vi "Display3DTest.vi"(8 "error in":errorcluster, 11 "Local":T7={"Parameter"={"3D Plot"=[], "3D Scatter"=refnum, "Data"={"Split"={"X Train"=[], "X Test"=[], "Y Train"=[], "Y Test"=[]}, "Predict"=[]}, "Display"={"Choice"=enum."All", "Indexe"={"X"=0, "Y"=1, "Z"=2}}, "Point Property"={"Train Style"=enum."Full circle", "Test OK Style"=enum."Full square", "Label Color"=[8978528, 4367871, 1985280], "Test NO OK"={"Style"=enum."Cross", "Color"=16716800}}, "3D Plot Datatype.lvclass"=refnum}, "3DArray"=[], "Rating 3D Array"=[], "GoodPredict"=0, "Point ID"=[]}) -> (0 "error out":errorcluster, 3 "Local Out":T5={"Parameter"={"3D Plot"=[], "3D Scatter"=refnum, "Data"={"Split"={"X Train"=[], "X Test"=[], "Y Train"=[], "Y Test"=[]}, "Predict"=[]}, "Display"={"Choice"=enum."All", "Indexe"={"X"=0, "Y"=1, "Z"=2}}, "Point Property"={"Train Style"=enum."Full circle", "Test OK Style"=enum."Full square", "Label Color"=[8978528, 4367871, 1985280], "Test NO OK"={"Style"=enum."Cross", "Color"=16716800}}, "3D Plot Datatype.lvclass"=refnum}, "3DArray"=[], "Rating 3D Array"=[], "GoodPredict"=0, "Point ID"=[]})   [LabVIEW 2020]
doc: "Display the 3D predicted data"
uses:
  _Controls/3DParameters.ctl
  <vilib>/Math Plots/3D Math Plots/3D Plot/3D Plot Datatype/3D Plot Datatype.lvclass
  <vilib>/Math Plots/3D Math Plots/3D Scatter/3D Scatter XCtrl/3D Scatter.xctl
  _Controls/Datas.ctl
  _Controls/PointPropertyMultipleLabel.ctl
  _Controls/Style.ctl
  _Controls/3DData.ctl
  <vilib>/Math Plots/3D Math Plots/3D Plot/3D Plot/Typedef/Color Ramp Cluster.ctl
  <vilib>/Math Plots/3D Math Plots/3D Plot/3D Plot/3D Plot.lvclass
types:
  T1 = typedef "Datas.ctl" = cluster{"Split":cluster{"X Train":dbl[][], "X Test":dbl[][], "Y Train":dbl[][], "Y Test":dbl[][]}, "Predict":dbl[][]}
  T2 = typedef "PointPropertyMultipleLabel.ctl" = cluster{"Train Style":T3, "Test OK Style":T3, "Label Color":u32[], "Test NO OK":cluster{"Style":T3, "Color":u32}}
  T3 = typedef "Style.ctl" = enum16{"Empty circle", "Full circle", "Empty square", "Full square", "Cross"}
  T4 = typedef "3DData.ctl" = cluster{"Tag":i32, "X":dbl[], "Y":dbl[], "Z":dbl[]}
  T5 = cluster{"Parameter":cluster{"3D Plot":refnum<class "3D Plot Datatype.lvclass">[], "3D Scatter":refnum<vi>, "Data":T1, "Display":cluster{"Choice":enum16{"All", "Train", "Test"}, "Indexe":cluster{"X":i32, "Y":i32, "Z":i32}}, "Point Property":T2, "3D Plot Datatype.lvclass":refnum<class "3D Plot Datatype.lvclass">}, "3DArray":cluster{"X":dbl[], "Y":dbl[], "Z":dbl[]}[], "Rating 3D Array":T4[], "GoodPredict":i32, "Point ID":cluster{"DataUse":enum16{"Dataset", "Train", "Test"}, "Color":u32}[]}
  T6 = typedef "3DParameters.ctl" = cluster{"3D Plot":refnum<class "3D Plot Datatype.lvclass">[], "3D Scatter":refnum<vi>, "Data":T1, "Display":cluster{"Choice":enum16{"All", "Train", "Test"}, "Indexe":cluster{"X":i32, "Y":i32, "Z":i32}}, "Point Property":T2, "3D Plot Datatype.lvclass":refnum<class "3D Plot Datatype.lvclass">}
  T7 = cluster{"Parameter":T6, "3DArray":cluster{"X":dbl[], "Y":dbl[], "Z":dbl[]}[], "Rating 3D Array":T4[], "GoodPredict":i32, "Point ID":cluster{"DataUse":enum16{"Dataset", "Train", "Test"}, "Color":u32}[]}
  T8 = typedef "3D Plot.lvclass/Color Ramp Cluster.ctl" = cluster{"Color Ramp Style":enum16{"None", "Shaded", "Color spectrum", "Grey scale", "Custom"}, "Color Ramp Array":u32[], "Color Ramp Index":i32[], "Interpolate?":bool, "Logarithm?":bool}
  T9 = typedef "3D Plot.lvclass/Sprite Type.ctl" = enum16{"None", "Empty Square", "Solid Square", "Empty Diamond", "Solid Diamond", "Empty Circle", "Solid Circle", "Asterisk", "Bold X", "Wireframe Sphere", "Solid Sphere", "Wireframe Cube", "Solid Cube"}
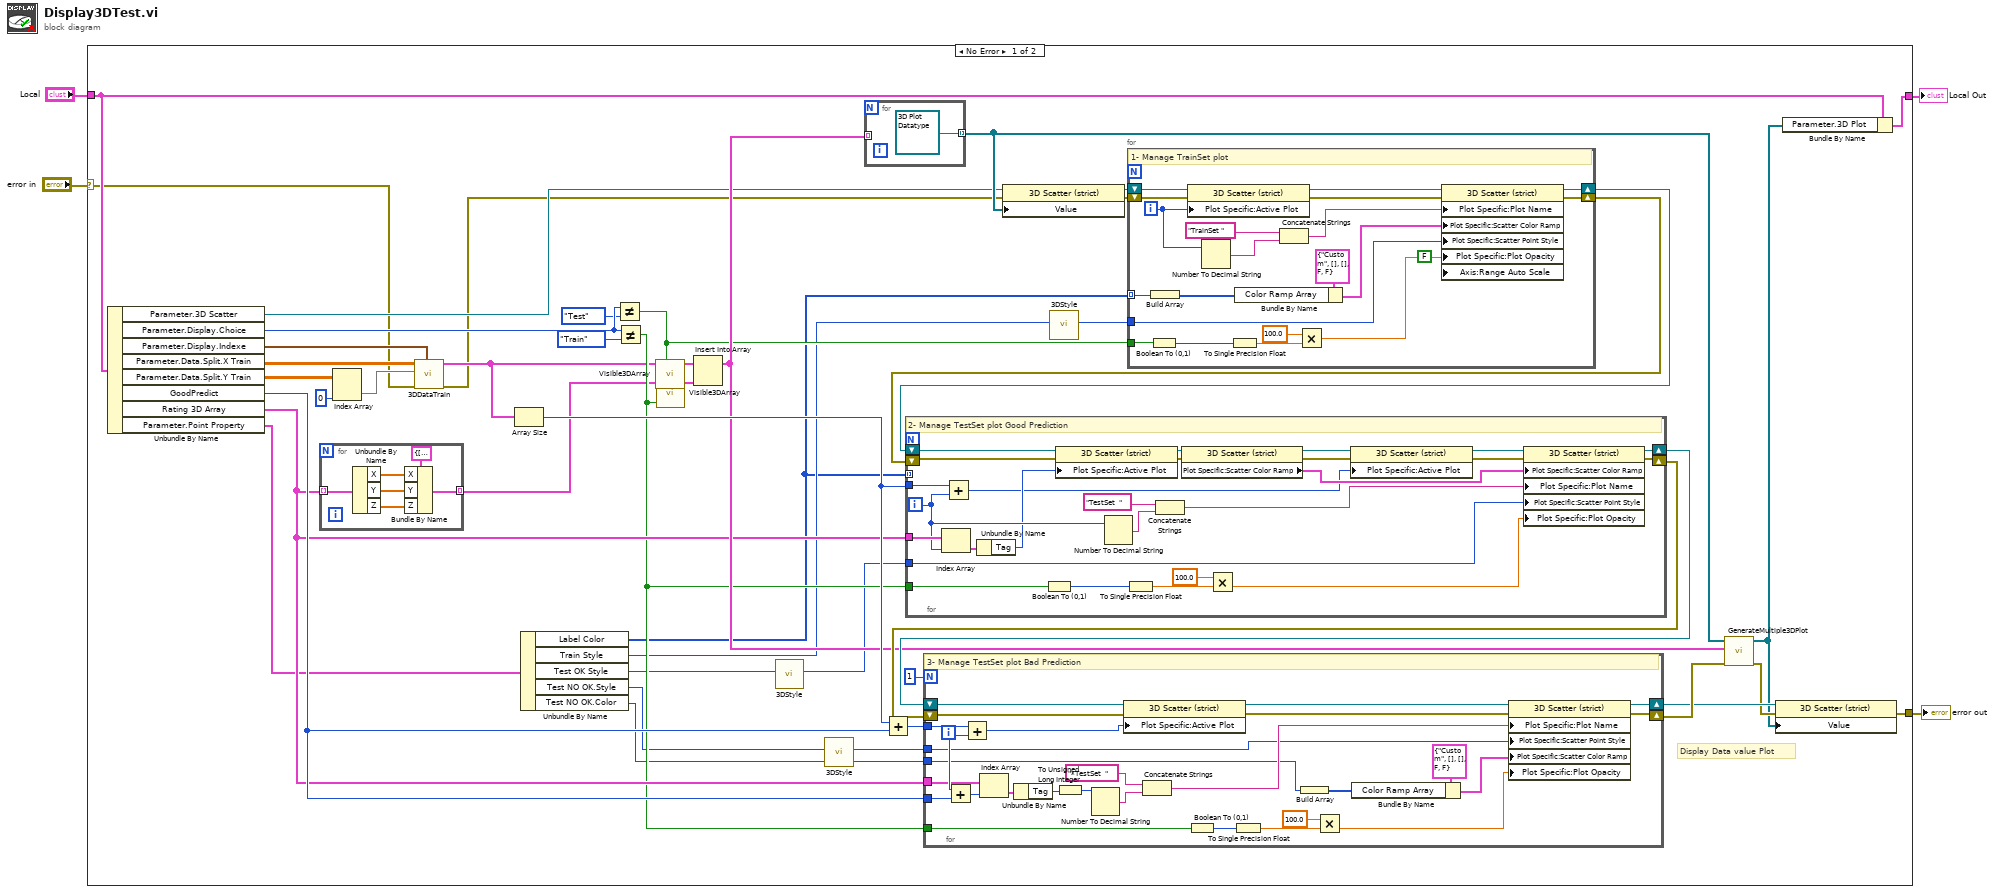
[diagram p0: block diagram]
diagram:
  n1 = case shown="No Error" "error in" {
    selector: "error in" -> [w15 w134]
    tunnel: [w28 w134] -> w3
    tunnel: "Local" -> [w39 w133]
    tunnel: [w38 w133] -> w1
    frame No Error {
      # "Display Data value Plot"
      n2 = Unbundle By Name(w39) -> ("Parameter.3D Scatter"=w32:refnum<vi>, "Parameter.Display.Choice"=w36:enum16{"All", "Train", "Test"}, "Parameter.Display.Indexe"=w16:cluster{"X":i32, "Y":i32, "Z":i32}, "Parameter.Data.Split.X Train"=w20:dbl[][], "Parameter.Data.Split.Y Train"=w35:dbl[][], "GoodPredict"=w34:i32, "Rating 3D Array"=w33:T4[], "Parameter.Point Property"=w14:T2)
      n3 = for {
        tunnel: w33 -> [w56] mode=indexing
        tunnel: [w54] -> w24 mode=indexing
        n4 = Unbundle By Name(w56) -> ("X"=w53:dbl[], "Y"=w52:dbl[], "Z"=w51:dbl[])
        n5 = Bundle By Name(cluster=cluster{"X":dbl[], "Y":dbl[], "Z":dbl[]} {"X"=[], "Y"=[], "Z"=[]} ("new element/subarray"), "X"=w53, "Y"=w52, "Z"=w51) -> (w54:cluster{"X":dbl[], "Y":dbl[], "Z":dbl[]})
      }
      n6 = Index Array(array=w35, index (col)=0 ("disabled index (col)")) -> (element=w19:dbl[])  [unwired: 1 in]
      n7 = call "3DDataTrain.vi"("Index"=w16, "error in"=w15, "Y"=w19, "X"=w20) -> ("error out"=w21:errorcluster, "3DArray"=w22:cluster{"X":dbl[], "Y":dbl[], "Z":dbl[]}[])  [unwired: 6 in]
      n8 = Array Size(array=w22) -> (size(s)=w42:i32)
      n9 = Unbundle By Name(w14) -> ("Label Color"=w8:u32[], "Train Style"=w10:T3, "Test OK Style"=w7:T3, "Test NO OK.Style"=w12:T3, "Test NO OK.Color"=w13:u32)
      n10 = Not Equal?(x=w36, y=enum16{"All", "Train", "Test"}."Test") -> (x != y?=w27:bool)
      n11 = Not Equal?(x=w36, y=enum16{"All", "Train", "Test"}."Train") -> (x != y?=w25:bool)
      n12 = call "Visible3DArray.vi"("Visible"=w27, "Array In"=w22) -> ("Array Out"=w26:cluster{"X":dbl[], "Y":dbl[], "Z":dbl[]}[])  [unwired: 9 in]
      n13 = call "Visible3DArray.vi"("Visible"=w25, "Array In"=w24) -> ("Array Out"=w23:cluster{"X":dbl[], "Y":dbl[], "Z":dbl[]}[])  [unwired: 9 in]
      n14 = Insert Into Array(array=w26, new element=w23) -> (w41:cluster{"X":dbl[], "Y":dbl[], "Z":dbl[]}[])  [unwired: 1 in]
      n15 = call "3DStyle.vi"("Style"=w7) -> ("Scatter Point Style"=w6:T9)  [unwired: 10 in]
      n16 = call "3DStyle.vi"("Style"=w12) -> ("Scatter Point Style"=w11:T9)  [unwired: 10 in]
      n17 = for {
        tunnel: w41 -> [_] mode=indexing
        tunnel: [refnum<class "3D Plot Datatype.lvclass"> refnum ("3D Plot Datatype.lvclass")] -> w37 mode=indexing
      }
      n18 = Add(x=w42, y=w34) -> (x+y=w46:i32)
      n19 = property class="3D Scatter (strict)"(reference=w32, error in=w21, "Value"=w37) -> (reference out=w44:refnum<vi>, error out=w43:errorcluster)
      n20 = call "3DStyle.vi"("Style"=w10) -> ("Scatter Point Style"=w9:T9)  [unwired: 10 in]
      n21 = for {
        shift-right: [w126] -> w50
        shift-left: w43 -> [w131]
        shift-right: [w125] -> w49
        shift-left: w44 -> [w132]
        tunnel: w27 -> [w123]
        tunnel: w8 -> [w115] mode=indexing
        tunnel: w9 -> [w112]
        i -> [w124]
        # "1- Manage TrainSet plot"
        n22 = Boolean To (0,1)(Boolean=w123) -> (0, 1=w122:i16)
        n23 = Build Array(w115) -> (w114:u32[])
        n24 = property class="3D Scatter (strict)"(reference=w132, error in=w131, "Plot Specific:Active Plot"=w124) -> (reference out=w130:refnum<vi>, error out=w129:errorcluster)
        n25 = Number To Decimal String(number=w124) -> (decimal integer string=w127:string)  [unwired: 1 in]
        n26 = To Single Precision Float(number=w122) -> (single precision float=w121:sgl)
        n27 = Bundle By Name(cluster=T8 {"Color Ramp Style"=enum."Custom", "Color Ramp Array"=[], "Color Ramp Index"=[], "Interpolate?"=FALSE, "Logarithm?"=FALSE} ("Spécifique à un tracé:Nuage:Rampe de couleur du nuage"), "Color Ramp Array"=w114) -> (w113:T8)
        n28 = Concatenate Strings("TrainSet " ("Plot.Plot Name"), w127) -> (w116:string)
        n29 = Multiply(x=sgl 100.0, y=w121) -> (x*y=w120:sgl)
        n30 = property class="3D Scatter (strict)"(reference=w130, error in=w129, "Plot Specific:Plot Name"=w116, "Plot Specific:Scatter Color Ramp"=w113, "Plot Specific:Scatter Point Style"=w112, "Plot Specific:Plot Opacity"=w120, "Axis:Range Auto Scale"=FALSE ("Axis:Range:Range Auto Scale")) -> (reference out=w125:refnum<vi>, error out=w126:errorcluster)
      }
      n31 = for {
        shift-right: [w68] -> w47
        shift-left: w50 -> [w73]
        shift-right: [w78] -> w48
        shift-left: w49 -> [w74]
        tunnel: w42 -> [w76]
        tunnel: w33 -> [w77]
        tunnel: w25 -> [w61]
        tunnel: w8 -> [_] mode=indexing
        tunnel: w6 -> [w57]
        i -> [w67]
        # "2- Manage TestSet plot Good Prediction"
        n32 = Index Array(array=w77, index=w67) -> (element=w75:T4)
        n33 = Add(x=w76, y=w67) -> (x+y=w63:i32)
        n34 = Unbundle By Name(w75) -> ("Tag"=w64:i32)
        n35 = Boolean To (0,1)(Boolean=w61) -> (0, 1=w62:i16)
        n36 = property class="3D Scatter (strict)"(reference=w74, error in=w73, "Plot Specific:Active Plot"=w64) -> (reference out=w72:refnum<vi>, error out=w71:errorcluster)
        n37 = Number To Decimal String(number=w67) -> (decimal integer string=w79:string)  [unwired: 1 in]
        n38 = To Single Precision Float(number=w62) -> (single precision float=w60:sgl)
        n39 = Concatenate Strings("TestSet  " ("Plot.Plot Name"), w79) -> (w66:string)
        n40 = property class="3D Scatter (strict)"(reference=w72, error in=w71) -> (reference out=w70:refnum<vi>, error out=w69:errorcluster, "Plot Specific:Scatter Color Ramp"=w65:T8)
        n41 = Multiply(x=sgl 100.0, y=w60) -> (x*y=w59:sgl)
        n42 = property class="3D Scatter (strict)"(reference=w70, error in=w69, "Plot Specific:Active Plot"=w63) -> (reference out=w82:refnum<vi>, error out=w81:errorcluster)
        n43 = property class="3D Scatter (strict)"(reference=w82, error in=w81, "Plot Specific:Scatter Color Ramp"=w65, "Plot Specific:Plot Name"=w66, "Plot Specific:Scatter Point Style"=w57, "Plot Specific:Plot Opacity"=w59) -> (reference out=w78:refnum<vi>, error out=w68:errorcluster)
      }
      n44 = for {
        N: 1 -> [_]
        shift-right: [w102] -> w40
        shift-left: w47 -> [w96]
        shift-right: [w106] -> w31
        shift-left: w48 -> [w95]
        tunnel: w46 -> [w105]
        tunnel: w33 -> [w99]
        tunnel: w34 -> [w100]
        tunnel: w25 -> [w90]
        tunnel: w13 -> [w84]
        tunnel: w11 -> [w83]
        i -> [w101]
        # "3- Manage TestSet plot Bad Prediction"
        n45 = Add(x=w101, y=w100) -> (x+y=w98:i32)
        n46 = Add(x=w105, y=w101) -> (x+y=w94:i32)
        n47 = Index Array(array=w99, index=w98) -> (element=w104:T4)
        n48 = Unbundle By Name(w104) -> ("Tag"=w103:i32)
        n49 = To Unsigned Long Integer(number=w103) -> (unsigned 32bit integer=w97:u32)
        n50 = Number To Decimal String(number=w97) -> (decimal integer string=w107:string)  [unwired: 1 in]
        n51 = property class="3D Scatter (strict)"(reference=w95, error in=w96, "Plot Specific:Active Plot"=w94) -> (reference out=w110:refnum<vi>, error out=w109:errorcluster)
        n52 = Concatenate Strings("*TestSet  " ("Plot.Plot Name"), w107) -> (w93:string)
        n53 = Boolean To (0,1)(Boolean=w90) -> (0, 1=w91:i16)
        n54 = To Single Precision Float(number=w91) -> (single precision float=w89:sgl)
        n55 = Build Array(w84) -> (w85:u32[])
        n56 = Multiply(x=sgl 100.0, y=w89) -> (x*y=w88:sgl)
        n57 = Bundle By Name(cluster=T8 {"Color Ramp Style"=enum."Custom", "Color Ramp Array"=[], "Color Ramp Index"=[], "Interpolate?"=FALSE, "Logarithm?"=FALSE} ("Spécifique à un tracé:Nuage:Rampe de couleur du nuage"), "Color Ramp Array"=w85) -> (w92:T8)
        n58 = property class="3D Scatter (strict)"(reference=w110, error in=w109, "Plot Specific:Plot Name"=w93, "Plot Specific:Scatter Point Style"=w83, "Plot Specific:Scatter Color Ramp"=w92, "Plot Specific:Plot Opacity"=w88) -> (reference out=w106:refnum<vi>, error out=w102:errorcluster)
      }
      n59 = call "GenerateMultiple3DPlot.vi"("error in"=w40, "3D Array"=w41, "3D Scatter"=w37) -> ("error out"=w30:errorcluster, "3D Scatter Out"=w29:refnum<class "3D Plot Datatype.lvclass">[])  [unwired: 7 in]
      n60 = property class="3D Scatter (strict)"(reference=w31, error in=w30, "Value"=w29) -> (error out=w28:errorcluster)  [unwired: 1 out]
      n61 = Bundle By Name(cluster=w39, "Parameter.3D Plot"=w29) -> (w38:T7)
    }
    frame Error {
    }
  }
  "error out" <- w3
  "Local Out" <- w1
